vi "all vis.vi"   [LabVIEW 2015]
uses:
  xlsxwriter.lvlib
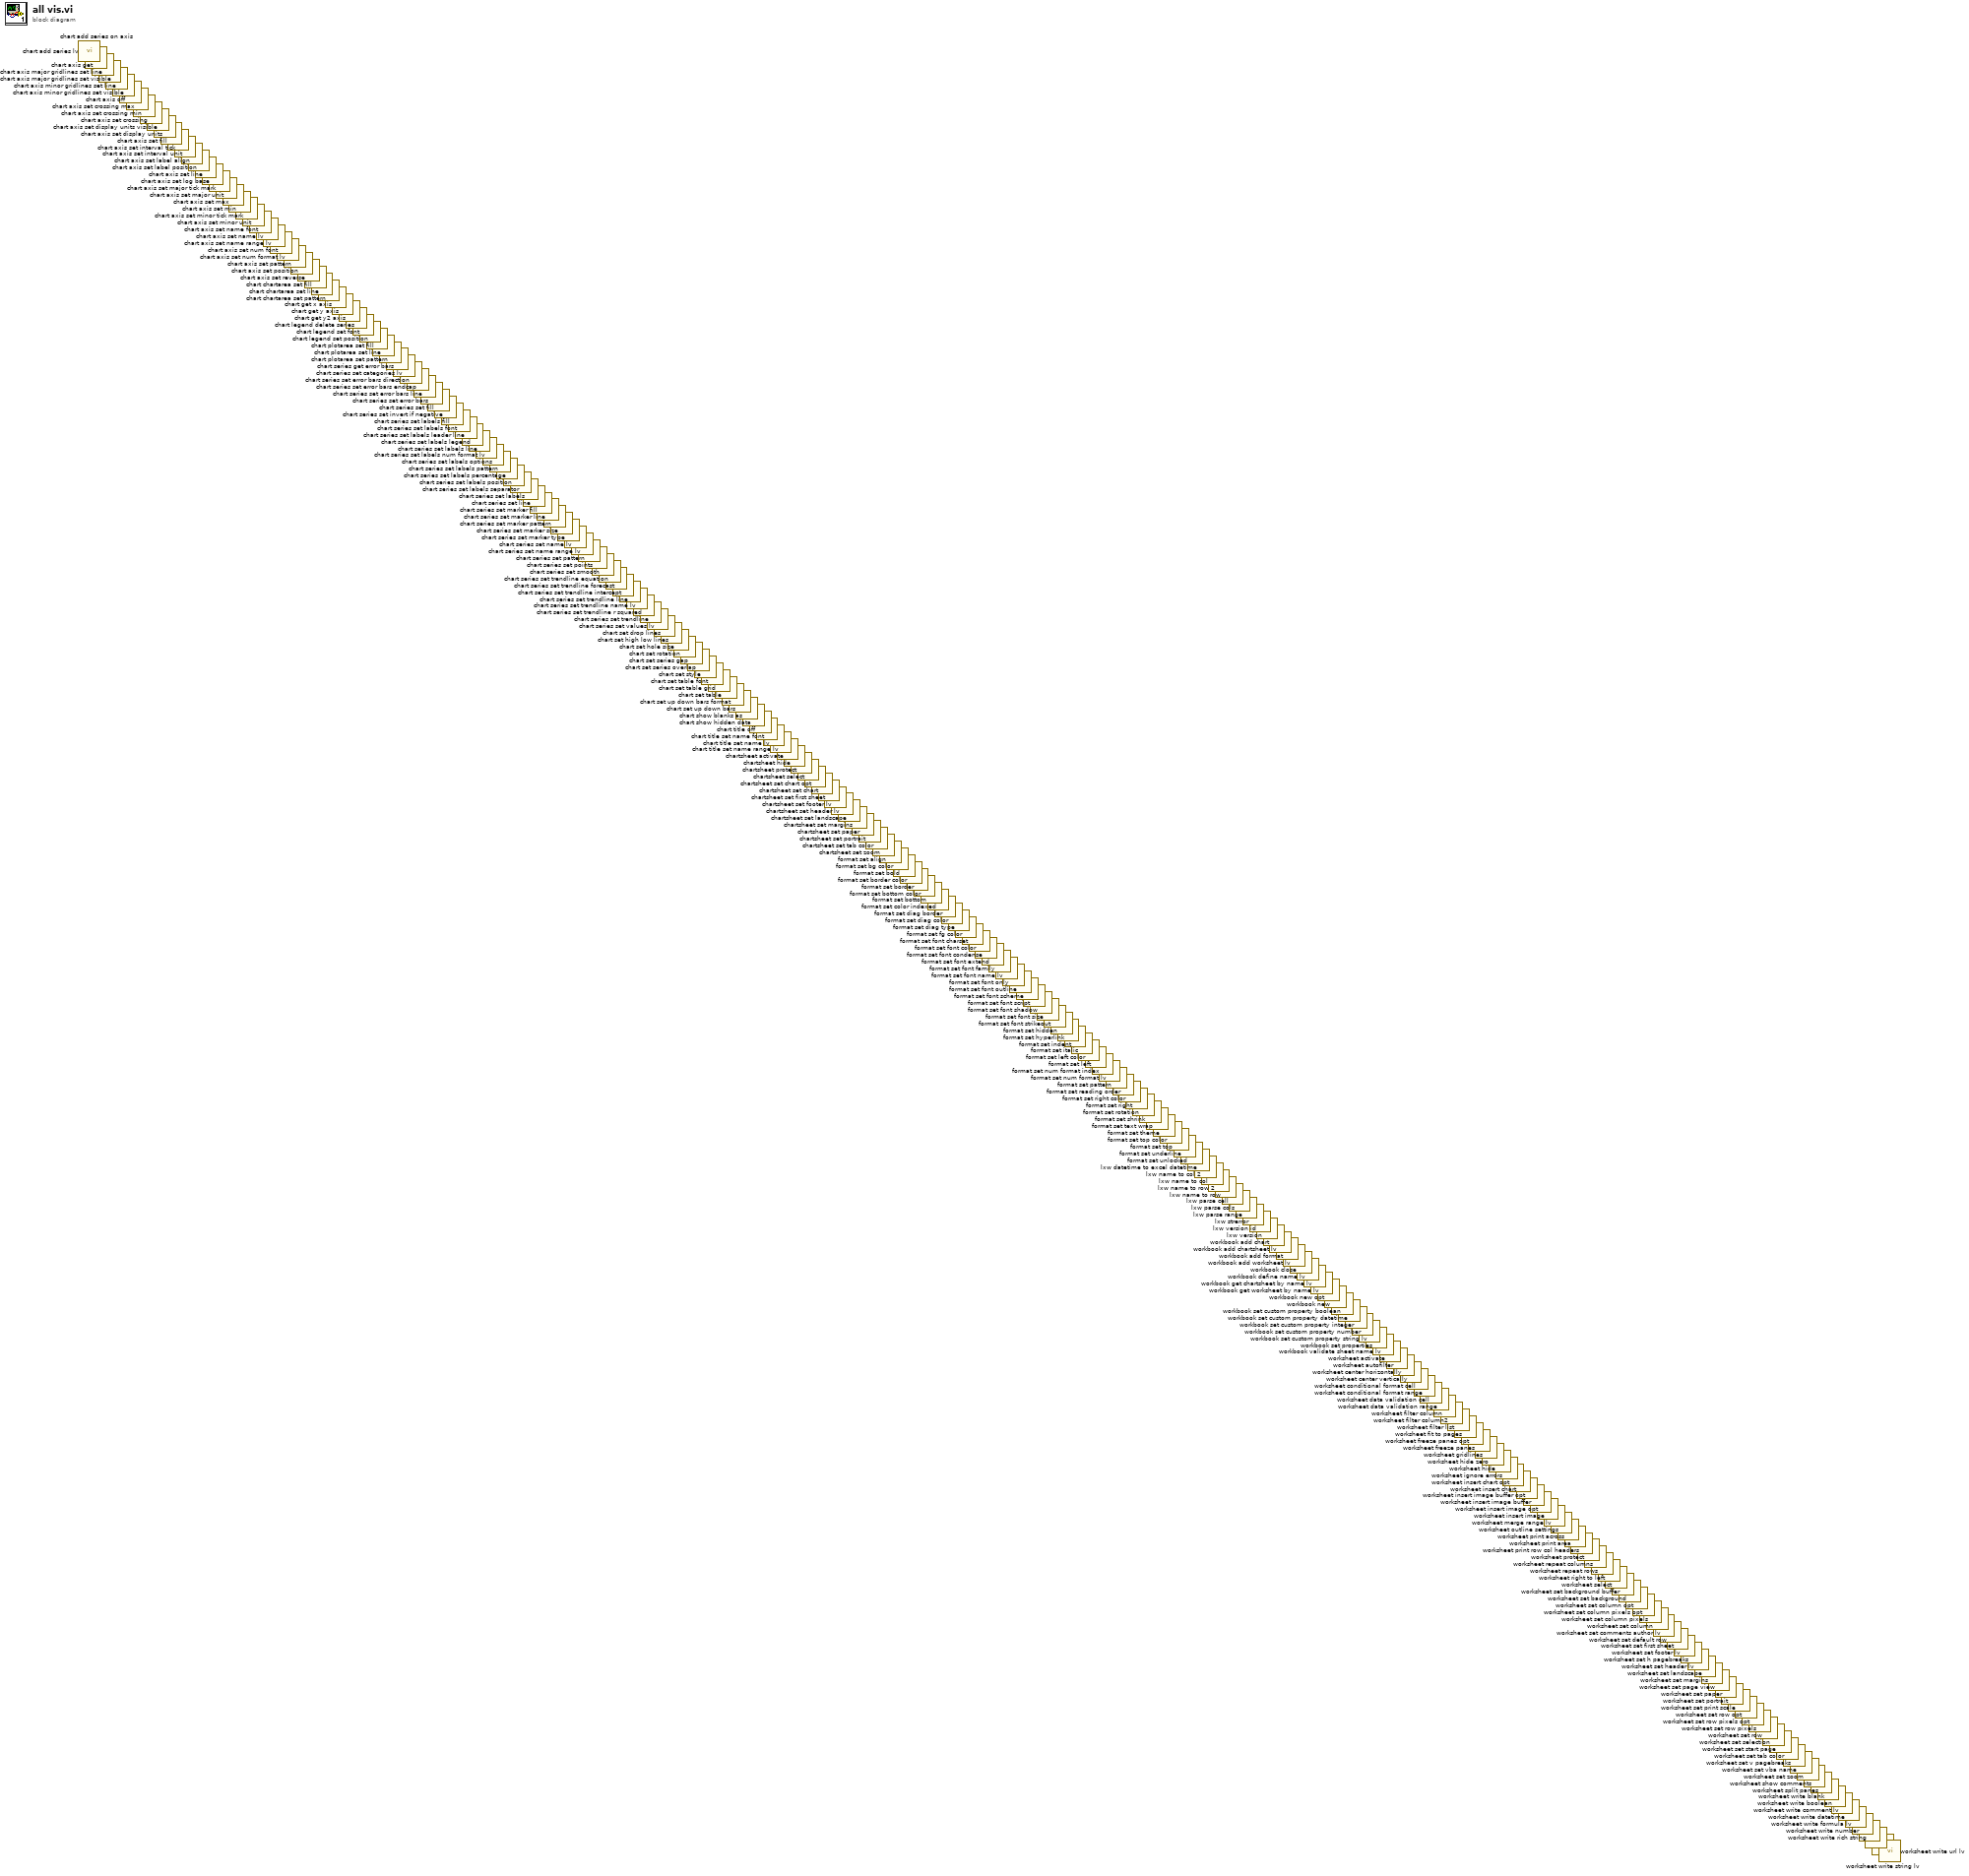
[diagram p0: block diagram]
diagram:
  n1 = call "chart add series lv.vi"() -> ()  [unwired: 10 in, 2 out]
  n2 = call "chart add series on axis.vi"() -> ()  [unwired: 10 in, 2 out]
  n3 = call "chart axis get.vi"() -> ()  [unwired: 10 in, 2 out]
  n4 = call "chart axis major gridlines set line.vi"() -> ()  [unwired: 10 in, 2 out]
  n5 = call "chart axis major gridlines set visible.vi"() -> ()  [unwired: 11 in, 1 out]
  n6 = call "chart axis minor gridlines set line.vi"() -> ()  [unwired: 10 in, 2 out]
  n7 = call "chart axis minor gridlines set visible.vi"() -> ()  [unwired: 11 in, 1 out]
  n8 = call "chart axis off.vi"() -> ()  [unwired: 11 in, 1 out]
  n9 = call "chart axis set crossing max.vi"() -> ()  [unwired: 11 in, 1 out]
  n10 = call "chart axis set crossing min.vi"() -> ()  [unwired: 11 in, 1 out]
  n11 = call "chart axis set crossing.vi"() -> ()  [unwired: 11 in, 1 out]
  n12 = call "chart axis set display units visible.vi"() -> ()  [unwired: 11 in, 1 out]
  n13 = call "chart axis set display units.vi"() -> ()  [unwired: 11 in, 1 out]
  n14 = call "chart axis set fill.vi"() -> ()  [unwired: 10 in, 2 out]
  n15 = call "chart axis set interval tick.vi"() -> ()  [unwired: 11 in, 1 out]
  n16 = call "chart axis set interval unit.vi"() -> ()  [unwired: 11 in, 1 out]
  n17 = call "chart axis set label align.vi"() -> ()  [unwired: 11 in, 1 out]
  n18 = call "chart axis set label position.vi"() -> ()  [unwired: 11 in, 1 out]
  n19 = call "chart axis set line.vi"() -> ()  [unwired: 10 in, 2 out]
  n20 = call "chart axis set log base.vi"() -> ()  [unwired: 11 in, 1 out]
  n21 = call "chart axis set major tick mark.vi"() -> ()  [unwired: 11 in, 1 out]
  n22 = call "chart axis set major unit.vi"() -> ()  [unwired: 11 in, 1 out]
  n23 = call "chart axis set max.vi"() -> ()  [unwired: 11 in, 1 out]
  n24 = call "chart axis set min.vi"() -> ()  [unwired: 11 in, 1 out]
  n25 = call "chart axis set minor tick mark.vi"() -> ()  [unwired: 11 in, 1 out]
  n26 = call "chart axis set minor unit.vi"() -> ()  [unwired: 11 in, 1 out]
  n27 = call "chart axis set name font.vi"() -> ()  [unwired: 10 in, 2 out]
  n28 = call "chart axis set name lv.vi"() -> ()  [unwired: 11 in, 1 out]
  n29 = call "chart axis set name range lv.vi"() -> ()  [unwired: 11 in, 1 out]
  n30 = call "chart axis set num font.vi"() -> ()  [unwired: 10 in, 2 out]
  n31 = call "chart axis set num format lv.vi"() -> ()  [unwired: 11 in, 1 out]
  n32 = call "chart axis set pattern.vi"() -> ()  [unwired: 10 in, 2 out]
  n33 = call "chart axis set position.vi"() -> ()  [unwired: 11 in, 1 out]
  n34 = call "chart axis set reverse.vi"() -> ()  [unwired: 11 in, 1 out]
  n35 = call "chart chartarea set fill.vi"() -> ()  [unwired: 10 in, 2 out]
  n36 = call "chart chartarea set line.vi"() -> ()  [unwired: 10 in, 2 out]
  n37 = call "chart chartarea set pattern.vi"() -> ()  [unwired: 10 in, 2 out]
  n38 = call "chart get x axis.vi"() -> ()  [unwired: 10 in, 2 out]
  n39 = call "chart get y axis.vi"() -> ()  [unwired: 10 in, 2 out]
  n40 = call "chart get y2 axis.vi"() -> ()  [unwired: 10 in, 2 out]
  n41 = call "chart legend delete series.vi"() -> ()  [unwired: 10 in, 2 out]
  n42 = call "chart legend set font.vi"() -> ()  [unwired: 10 in, 2 out]
  n43 = call "chart legend set position.vi"() -> ()  [unwired: 11 in, 1 out]
  n44 = call "chart plotarea set fill.vi"() -> ()  [unwired: 10 in, 2 out]
  n45 = call "chart plotarea set line.vi"() -> ()  [unwired: 10 in, 2 out]
  n46 = call "chart plotarea set pattern.vi"() -> ()  [unwired: 10 in, 2 out]
  n47 = call "chart series get error bars.vi"() -> ()  [unwired: 10 in, 2 out]
  n48 = call "chart series set categories lv.vi"() -> ()  [unwired: 11 in, 1 out]
  n49 = call "chart series set error bars direction.vi"() -> ()  [unwired: 11 in, 1 out]
  n50 = call "chart series set error bars endcap.vi"() -> ()  [unwired: 11 in, 1 out]
  n51 = call "chart series set error bars line.vi"() -> ()  [unwired: 10 in, 2 out]
  n52 = call "chart series set error bars.vi"() -> ()  [unwired: 11 in, 1 out]
  n53 = call "chart series set fill.vi"() -> ()  [unwired: 10 in, 2 out]
  n54 = call "chart series set invert if negative.vi"() -> ()  [unwired: 11 in, 1 out]
  n55 = call "chart series set labels fill.vi"() -> ()  [unwired: 10 in, 2 out]
  n56 = call "chart series set labels font.vi"() -> ()  [unwired: 10 in, 2 out]
  n57 = call "chart series set labels leader line.vi"() -> ()  [unwired: 11 in, 1 out]
  n58 = call "chart series set labels legend.vi"() -> ()  [unwired: 11 in, 1 out]
  n59 = call "chart series set labels line.vi"() -> ()  [unwired: 10 in, 2 out]
  n60 = call "chart series set labels num format lv.vi"() -> ()  [unwired: 11 in, 1 out]
  n61 = call "chart series set labels options.vi"() -> ()  [unwired: 11 in, 1 out]
  n62 = call "chart series set labels pattern.vi"() -> ()  [unwired: 10 in, 2 out]
  n63 = call "chart series set labels percentage.vi"() -> ()  [unwired: 11 in, 1 out]
  n64 = call "chart series set labels position.vi"() -> ()  [unwired: 11 in, 1 out]
  n65 = call "chart series set labels separator.vi"() -> ()  [unwired: 11 in, 1 out]
  n66 = call "chart series set labels.vi"() -> ()  [unwired: 11 in, 1 out]
  n67 = call "chart series set line.vi"() -> ()  [unwired: 10 in, 2 out]
  n68 = call "chart series set marker fill.vi"() -> ()  [unwired: 10 in, 2 out]
  n69 = call "chart series set marker line.vi"() -> ()  [unwired: 10 in, 2 out]
  n70 = call "chart series set marker pattern.vi"() -> ()  [unwired: 10 in, 2 out]
  n71 = call "chart series set marker size.vi"() -> ()  [unwired: 11 in, 1 out]
  n72 = call "chart series set marker type.vi"() -> ()  [unwired: 11 in, 1 out]
  n73 = call "chart series set name lv.vi"() -> ()  [unwired: 11 in, 1 out]
  n74 = call "chart series set name range lv.vi"() -> ()  [unwired: 11 in, 1 out]
  n75 = call "chart series set pattern.vi"() -> ()  [unwired: 10 in, 2 out]
  n76 = call "chart series set points.vi"() -> ()  [unwired: 11 in, 1 out]
  n77 = call "chart series set smooth.vi"() -> ()  [unwired: 11 in, 1 out]
  n78 = call "chart series set trendline equation.vi"() -> ()  [unwired: 10 in, 2 out]
  n79 = call "chart series set trendline forecast.vi"() -> ()  [unwired: 10 in, 2 out]
  n80 = call "chart series set trendline intercept.vi"() -> ()  [unwired: 10 in, 2 out]
  n81 = call "chart series set trendline line.vi"() -> ()  [unwired: 9 in, 3 out]
  n82 = call "chart series set trendline name lv.vi"() -> ()  [unwired: 11 in, 1 out]
  n83 = call "chart series set trendline r squared.vi"() -> ()  [unwired: 10 in, 2 out]
  n84 = call "chart series set trendline.vi"() -> ()  [unwired: 10 in, 2 out]
  n85 = call "chart series set values lv.vi"() -> ()  [unwired: 11 in, 1 out]
  n86 = call "chart set drop lines.vi"() -> ()  [unwired: 10 in, 2 out]
  n87 = call "chart set high low lines.vi"() -> ()  [unwired: 10 in, 2 out]
  n88 = call "chart set hole size.vi"() -> ()  [unwired: 11 in, 1 out]
  n89 = call "chart set rotation.vi"() -> ()  [unwired: 11 in, 1 out]
  n90 = call "chart set series gap.vi"() -> ()  [unwired: 11 in, 1 out]
  n91 = call "chart set series overlap.vi"() -> ()  [unwired: 11 in, 1 out]
  n92 = call "chart set style.vi"() -> ()  [unwired: 11 in, 1 out]
  n93 = call "chart set table font.vi"() -> ()  [unwired: 10 in, 2 out]
  n94 = call "chart set table grid.vi"() -> ()  [unwired: 11 in, 1 out]
  n95 = call "chart set table.vi"() -> ()  [unwired: 11 in, 1 out]
  n96 = call "chart set up down bars format.vi"() -> ()  [unwired: 11 in, 5 out]
  n97 = call "chart set up down bars.vi"() -> ()  [unwired: 11 in, 1 out]
  n98 = call "chart show blanks as.vi"() -> ()  [unwired: 11 in, 1 out]
  n99 = call "chart show hidden data.vi"() -> ()  [unwired: 11 in, 1 out]
  n100 = call "chart title off.vi"() -> ()  [unwired: 11 in, 1 out]
  n101 = call "chart title set name font.vi"() -> ()  [unwired: 10 in, 2 out]
  n102 = call "chart title set name lv.vi"() -> ()  [unwired: 11 in, 1 out]
  n103 = call "chart title set name range lv.vi"() -> ()  [unwired: 11 in, 1 out]
  n104 = call "chartsheet activate.vi"() -> ()  [unwired: 11 in, 1 out]
  n105 = call "chartsheet hide.vi"() -> ()  [unwired: 11 in, 1 out]
  n106 = call "chartsheet protect.vi"() -> ()  [unwired: 10 in, 2 out]
  n107 = call "chartsheet select.vi"() -> ()  [unwired: 11 in, 1 out]
  n108 = call "chartsheet set chart opt.vi"() -> ()  [unwired: 9 in, 3 out]
  n109 = call "chartsheet set chart.vi"() -> ()  [unwired: 10 in, 2 out]
  n110 = call "chartsheet set first sheet.vi"() -> ()  [unwired: 11 in, 1 out]
  n111 = call "chartsheet set footer lv.vi"() -> ()  [unwired: 10 in, 2 out]
  n112 = call "chartsheet set header lv.vi"() -> ()  [unwired: 10 in, 2 out]
  n113 = call "chartsheet set landscape.vi"() -> ()  [unwired: 11 in, 1 out]
  n114 = call "chartsheet set margins.vi"() -> ()  [unwired: 11 in, 1 out]
  n115 = call "chartsheet set paper.vi"() -> ()  [unwired: 11 in, 1 out]
  n116 = call "chartsheet set portrait.vi"() -> ()  [unwired: 11 in, 1 out]
  n117 = call "chartsheet set tab color.vi"() -> ()  [unwired: 11 in, 1 out]
  n118 = call "chartsheet set zoom.vi"() -> ()  [unwired: 11 in, 1 out]
  n119 = call "format set align.vi"() -> ()  [unwired: 11 in, 1 out]
  n120 = call "format set bg color.vi"() -> ()  [unwired: 11 in, 1 out]
  n121 = call "format set bold.vi"() -> ()  [unwired: 11 in, 1 out]
  n122 = call "format set border color.vi"() -> ()  [unwired: 11 in, 1 out]
  n123 = call "format set border.vi"() -> ()  [unwired: 11 in, 1 out]
  n124 = call "format set bottom color.vi"() -> ()  [unwired: 11 in, 1 out]
  n125 = call "format set bottom.vi"() -> ()  [unwired: 11 in, 1 out]
  n126 = call "format set color indexed.vi"() -> ()  [unwired: 11 in, 1 out]
  n127 = call "format set diag border.vi"() -> ()  [unwired: 11 in, 1 out]
  n128 = call "format set diag color.vi"() -> ()  [unwired: 11 in, 1 out]
  n129 = call "format set diag type.vi"() -> ()  [unwired: 11 in, 1 out]
  n130 = call "format set fg color.vi"() -> ()  [unwired: 11 in, 1 out]
  n131 = call "format set font charset.vi"() -> ()  [unwired: 11 in, 1 out]
  n132 = call "format set font color.vi"() -> ()  [unwired: 11 in, 1 out]
  n133 = call "format set font condense.vi"() -> ()  [unwired: 11 in, 1 out]
  n134 = call "format set font extend.vi"() -> ()  [unwired: 11 in, 1 out]
  n135 = call "format set font family.vi"() -> ()  [unwired: 11 in, 1 out]
  n136 = call "format set font name lv.vi"() -> ()  [unwired: 11 in, 1 out]
  n137 = call "format set font only.vi"() -> ()  [unwired: 11 in, 1 out]
  n138 = call "format set font outline.vi"() -> ()  [unwired: 11 in, 1 out]
  n139 = call "format set font scheme.vi"() -> ()  [unwired: 11 in, 1 out]
  n140 = call "format set font script.vi"() -> ()  [unwired: 11 in, 1 out]
  n141 = call "format set font shadow.vi"() -> ()  [unwired: 11 in, 1 out]
  n142 = call "format set font size.vi"() -> ()  [unwired: 11 in, 1 out]
  n143 = call "format set font strikeout.vi"() -> ()  [unwired: 11 in, 1 out]
  n144 = call "format set hidden.vi"() -> ()  [unwired: 11 in, 1 out]
  n145 = call "format set hyperlink.vi"() -> ()  [unwired: 11 in, 1 out]
  n146 = call "format set indent.vi"() -> ()  [unwired: 11 in, 1 out]
  n147 = call "format set italic.vi"() -> ()  [unwired: 11 in, 1 out]
  n148 = call "format set left color.vi"() -> ()  [unwired: 11 in, 1 out]
  n149 = call "format set left.vi"() -> ()  [unwired: 11 in, 1 out]
  n150 = call "format set num format index.vi"() -> ()  [unwired: 11 in, 1 out]
  n151 = call "format set num format lv.vi"() -> ()  [unwired: 11 in, 1 out]
  n152 = call "format set pattern.vi"() -> ()  [unwired: 11 in, 1 out]
  n153 = call "format set reading order.vi"() -> ()  [unwired: 11 in, 1 out]
  n154 = call "format set right color.vi"() -> ()  [unwired: 11 in, 1 out]
  n155 = call "format set right.vi"() -> ()  [unwired: 11 in, 1 out]
  n156 = call "format set rotation.vi"() -> ()  [unwired: 11 in, 1 out]
  n157 = call "format set shrink.vi"() -> ()  [unwired: 11 in, 1 out]
  n158 = call "format set text wrap.vi"() -> ()  [unwired: 11 in, 1 out]
  n159 = call "format set theme.vi"() -> ()  [unwired: 11 in, 1 out]
  n160 = call "format set top color.vi"() -> ()  [unwired: 11 in, 1 out]
  n161 = call "format set top.vi"() -> ()  [unwired: 11 in, 1 out]
  n162 = call "format set underline.vi"() -> ()  [unwired: 11 in, 1 out]
  n163 = call "format set unlocked.vi"() -> ()  [unwired: 11 in, 1 out]
  n164 = call "lxw datetime to excel datetime.vi"() -> ()  [unwired: 9 in, 3 out]
  n165 = call "lxw name to col 2.vi"() -> ()  [unwired: 10 in, 2 out]
  n166 = call "lxw name to col.vi"() -> ()  [unwired: 10 in, 2 out]
  n167 = call "lxw name to row 2.vi"() -> ()  [unwired: 10 in, 2 out]
  n168 = call "lxw name to row.vi"() -> ()  [unwired: 10 in, 2 out]
  n169 = call "lxw parse cell.vi"() -> ()  [unwired: 9 in, 3 out]
  n170 = call "lxw parse cols.vi"() -> ()  [unwired: 9 in, 3 out]
  n171 = call "lxw parse range.vi"() -> ()  [unwired: 11 in, 5 out]
  n172 = call "lxw strerror.vi"() -> ()  [unwired: 10 in, 2 out]
  n173 = call "lxw version id.vi"() -> ()  [unwired: 10 in, 2 out]
  n174 = call "lxw version.vi"() -> ()  [unwired: 11 in, 1 out]
  n175 = call "workbook add chart.vi"() -> ()  [unwired: 10 in, 2 out]
  n176 = call "workbook add chartsheet lv.vi"() -> ()  [unwired: 10 in, 2 out]
  n177 = call "workbook add format.vi"() -> ()  [unwired: 10 in, 2 out]
  n178 = call "workbook add worksheet lv.vi"() -> ()  [unwired: 10 in, 2 out]
  n179 = call "workbook close.vi"() -> ()  [unwired: 10 in, 2 out]
  n180 = call "workbook define name lv.vi"() -> ()  [unwired: 10 in, 2 out]
  n181 = call "workbook get chartsheet by name lv.vi"() -> ()  [unwired: 10 in, 2 out]
  n182 = call "workbook get worksheet by name lv.vi"() -> ()  [unwired: 10 in, 2 out]
  n183 = call "workbook new opt.vi"() -> ()  [unwired: 10 in, 2 out]
  n184 = call "workbook new.vi"() -> ()  [unwired: 10 in, 2 out]
  n185 = call "workbook set custom property boolean.vi"() -> ()  [unwired: 10 in, 2 out]
  n186 = call "workbook set custom property datetime.vi"() -> ()  [unwired: 9 in, 3 out]
  n187 = call "workbook set custom property integer.vi"() -> ()  [unwired: 10 in, 2 out]
  n188 = call "workbook set custom property number.vi"() -> ()  [unwired: 10 in, 2 out]
  n189 = call "workbook set custom property string lv.vi"() -> ()  [unwired: 10 in, 2 out]
  n190 = call "workbook set properties.vi"() -> ()  [unwired: 10 in, 2 out]
  n191 = call "workbook validate sheet name lv.vi"() -> ()  [unwired: 10 in, 2 out]
  n192 = call "worksheet activate.vi"() -> ()  [unwired: 11 in, 1 out]
  n193 = call "worksheet autofilter.vi"() -> ()  [unwired: 10 in, 2 out]
  n194 = call "worksheet center horizontally.vi"() -> ()  [unwired: 11 in, 1 out]
  n195 = call "worksheet center vertically.vi"() -> ()  [unwired: 11 in, 1 out]
  n196 = call "worksheet conditional format cell.vi"() -> ()  [unwired: 10 in, 2 out]
  n197 = call "worksheet conditional format range.vi"() -> ()  [unwired: 10 in, 2 out]
  n198 = call "worksheet data validation cell.vi"() -> ()  [unwired: 10 in, 2 out]
  n199 = call "worksheet data validation range.vi"() -> ()  [unwired: 10 in, 2 out]
  n200 = call "worksheet filter column.vi"() -> ()  [unwired: 10 in, 2 out]
  n201 = call "worksheet filter column2.vi"() -> ()  [unwired: 10 in, 2 out]
  n202 = call "worksheet filter list.vi"() -> ()  [unwired: 10 in, 2 out]
  n203 = call "worksheet fit to pages.vi"() -> ()  [unwired: 11 in, 1 out]
  n204 = call "worksheet freeze panes opt.vi"() -> ()  [unwired: 10 in, 2 out]
  n205 = call "worksheet freeze panes.vi"() -> ()  [unwired: 10 in, 2 out]
  n206 = call "worksheet gridlines.vi"() -> ()  [unwired: 11 in, 1 out]
  n207 = call "worksheet hide zero.vi"() -> ()  [unwired: 11 in, 1 out]
  n208 = call "worksheet hide.vi"() -> ()  [unwired: 11 in, 1 out]
  n209 = call "worksheet ignore errors.vi"() -> ()  [unwired: 11 in, 1 out]
  n210 = call "worksheet insert chart opt.vi"() -> ()  [unwired: 9 in, 3 out]
  n211 = call "worksheet insert chart.vi"() -> ()  [unwired: 10 in, 2 out]
  n212 = call "worksheet insert image buffer opt.vi"() -> ()  [unwired: 9 in, 3 out]
  n213 = call "worksheet insert image buffer.vi"() -> ()  [unwired: 10 in, 2 out]
  n214 = call "worksheet insert image opt.vi"() -> ()  [unwired: 9 in, 3 out]
  n215 = call "worksheet insert image.vi"() -> ()  [unwired: 10 in, 2 out]
  n216 = call "worksheet merge range lv.vi"() -> ()  [unwired: 10 in, 2 out]
  n217 = call "worksheet outline settings.vi"() -> ()  [unwired: 11 in, 1 out]
  n218 = call "worksheet print across.vi"() -> ()  [unwired: 11 in, 1 out]
  n219 = call "worksheet print area.vi"() -> ()  [unwired: 10 in, 2 out]
  n220 = call "worksheet print row col headers.vi"() -> ()  [unwired: 11 in, 1 out]
  n221 = call "worksheet protect.vi"() -> ()  [unwired: 10 in, 2 out]
  n222 = call "worksheet repeat columns.vi"() -> ()  [unwired: 10 in, 2 out]
  n223 = call "worksheet repeat rows.vi"() -> ()  [unwired: 10 in, 2 out]
  n224 = call "worksheet right to left.vi"() -> ()  [unwired: 11 in, 1 out]
  n225 = call "worksheet select.vi"() -> ()  [unwired: 11 in, 1 out]
  n226 = call "worksheet set background buffer.vi"() -> ()  [unwired: 10 in, 2 out]
  n227 = call "worksheet set background.vi"() -> ()  [unwired: 10 in, 2 out]
  n228 = call "worksheet set column opt.vi"() -> ()  [unwired: 9 in, 3 out]
  n229 = call "worksheet set column pixels opt.vi"() -> ()  [unwired: 9 in, 3 out]
  n230 = call "worksheet set column pixels.vi"() -> ()  [unwired: 10 in, 2 out]
  n231 = call "worksheet set column.vi"() -> ()  [unwired: 10 in, 2 out]
  n232 = call "worksheet set comments author lv.vi"() -> ()  [unwired: 11 in, 1 out]
  n233 = call "worksheet set default row.vi"() -> ()  [unwired: 11 in, 1 out]
  n234 = call "worksheet set first sheet.vi"() -> ()  [unwired: 11 in, 1 out]
  n235 = call "worksheet set footer lv.vi"() -> ()  [unwired: 10 in, 2 out]
  n236 = call "worksheet set h pagebreaks.vi"() -> ()  [unwired: 11 in, 1 out]
  n237 = call "worksheet set header lv.vi"() -> ()  [unwired: 10 in, 2 out]
  n238 = call "worksheet set landscape.vi"() -> ()  [unwired: 11 in, 1 out]
  n239 = call "worksheet set margins.vi"() -> ()  [unwired: 11 in, 1 out]
  n240 = call "worksheet set page view.vi"() -> ()  [unwired: 11 in, 1 out]
  n241 = call "worksheet set paper.vi"() -> ()  [unwired: 11 in, 1 out]
  n242 = call "worksheet set portrait.vi"() -> ()  [unwired: 11 in, 1 out]
  n243 = call "worksheet set print scale.vi"() -> ()  [unwired: 11 in, 1 out]
  n244 = call "worksheet set row opt.vi"() -> ()  [unwired: 9 in, 3 out]
  n245 = call "worksheet set row pixels opt.vi"() -> ()  [unwired: 9 in, 3 out]
  n246 = call "worksheet set row pixels.vi"() -> ()  [unwired: 10 in, 2 out]
  n247 = call "worksheet set row.vi"() -> ()  [unwired: 10 in, 2 out]
  n248 = call "worksheet set selection.vi"() -> ()  [unwired: 11 in, 1 out]
  n249 = call "worksheet set start page.vi"() -> ()  [unwired: 11 in, 1 out]
  n250 = call "worksheet set tab color.vi"() -> ()  [unwired: 11 in, 1 out]
  n251 = call "worksheet set v pagebreaks.vi"() -> ()  [unwired: 11 in, 1 out]
  n252 = call "worksheet set vba name.vi"() -> ()  [unwired: 10 in, 2 out]
  n253 = call "worksheet set zoom.vi"() -> ()  [unwired: 11 in, 1 out]
  n254 = call "worksheet show comments.vi"() -> ()  [unwired: 11 in, 1 out]
  n255 = call "worksheet split panes.vi"() -> ()  [unwired: 10 in, 2 out]
  n256 = call "worksheet write blank.vi"() -> ()  [unwired: 10 in, 2 out]
  n257 = call "worksheet write boolean.vi"() -> ()  [unwired: 10 in, 2 out]
  n258 = call "worksheet write comment lv.vi"() -> ()  [unwired: 10 in, 2 out]
  n259 = call "worksheet write datetime.vi"() -> ()  [unwired: 9 in, 3 out]
  n260 = call "worksheet write formula lv.vi"() -> ()  [unwired: 10 in, 2 out]
  n261 = call "worksheet write number.vi"() -> ()  [unwired: 10 in, 2 out]
  n262 = call "worksheet write rich string.vi"() -> ()  [unwired: 10 in, 2 out]
  n263 = call "worksheet write string lv.vi"() -> ()  [unwired: 10 in, 2 out]
  n264 = call "worksheet write url lv.vi"() -> ()  [unwired: 10 in, 2 out]
